vi "Panther Dashboard--global.vi"() -> ()   [LabVIEW 2019]
panel:
  in  "Target":string
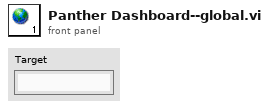
[diagram p1: front panel]
diagram:
